vi "DFD Plot Phase Delay.vi"(4 "phase delay unit":u16(ring) items=["Samples", "Seconds"], 5 "output option":u16(ring) items=["Auto", "Floating-Point Only", "Fixed-Point Only"], 6 "fs [Hz]":dbl=-1.0 format="%.2f", 7 "# freq bins":i32=-1, 8 "error in (no error)":errorcluster, 11 "filter in":T1={"mSRate_Fs"=1.0, "mSRate_Version"="2.0", "mSRate_Comments"="", "mSRate_OrgCoef"={"type"=enum."Undefined", "gain"=1.0, "coef a (k)"=[], "coef b (v)"=[]}, "mSRate_CurCoef"={"type"=enum."Undefined", "gain"=1.0, "coef a (k)"=[], "coef b (v)"=[]}, "mSRate_Quantized?"=FALSE, "mSRate_QCoef"={"type"=enum."Undefined", "gain"=1.0, "coef a (k)"=[], "coef b (v)"=[]}, "mSRate_QSettings"=[], "mSRate_Order"=0, "mSRate_Scaling"={"mSRate_ScaleByPowerOf2?"=FALSE, "mSRate_ScaleType"=enum."No Norm"}} {"mSRate_QSettings"."source" items=["Coef a/k"=0, "Coef b/v"=7, "Input"=1, "Output"=2, "Multiplicand"=3, "Product"=4, "Sum"=5, "Delay"=6, "Gain"=8]}) -> (0 "error out":errorcluster, 2 "phase delay":cluster{"f0":dbl, "df":dbl, "values":dbl[]}[](graph), 3 "filter out":T1={"mSRate_Fs"=1.0, "mSRate_Version"="2.0", "mSRate_Comments"="", "mSRate_OrgCoef"={"type"=enum."Undefined", "gain"=1.0, "coef a (k)"=[], "coef b (v)"=[]}, "mSRate_CurCoef"={"type"=enum."Undefined", "gain"=1.0, "coef a (k)"=[], "coef b (v)"=[]}, "mSRate_Quantized?"=FALSE, "mSRate_QCoef"={"type"=enum."Undefined", "gain"=1.0, "coef a (k)"=[], "coef b (v)"=[]}, "mSRate_QSettings"=[], "mSRate_Order"=0, "mSRate_Scaling"={"mSRate_ScaleByPowerOf2?"=FALSE, "mSRate_ScaleType"=enum."No Norm"}} {"mSRate_QSettings"."source" items=["Coef a/k"=0, "Coef b/v"=7, "Input"=1, "Output"=2, "Multiplicand"=3, "Product"=4, "Sum"=5, "Delay"=6, "Gain"=8]})   [LabVIEW 2017, in "NI_DigFilterLicensed.lvlib"]
doc: "Plots the phase delay response of a filter."
uses:
  <vilib>/addons/Digital Filter Design/NI_DigFilterLicensed.lvlib
  <vilib>/addons/Digital Filter Design/_Objects.llb/DFD Filter Obj.ctl
  <vilib>/addons/Digital Filter Design/_Objects.llb/DFD Filter Coef.ctl
  <vilib>/addons/Digital Filter Design/_Objects.llb/DFD Filter Structure Type Selector.ctl
  <vilib>/addons/Digital Filter Design/_Objects.llb/dfd_Internal Quantization Settings.ctl
  <vilib>/addons/Digital Filter Design/_Objects.llb/dfd_Internal Quantization Srcs.ctl
  <vilib>/addons/Digital Filter Design/_Objects.llb/DFD Coef Norm Type.ctl
  <vilib>/addons/Digital Filter Design/_Objects.llb/DFD Phase Setting.ctl
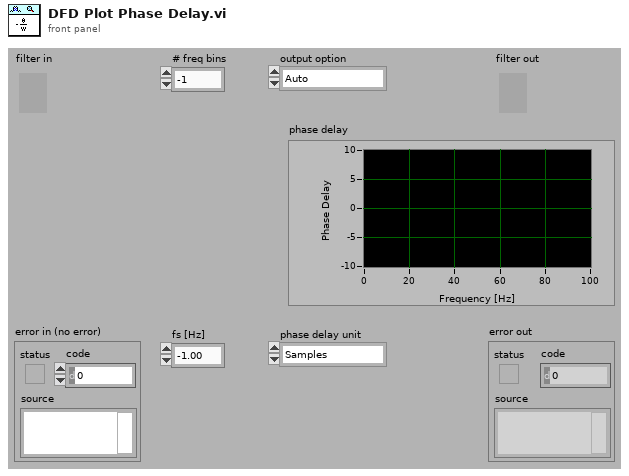
[diagram p1: front panel]
types:
  T1 = typedef "NI_DigFilterLicensed.lvlib/DFD Filter Obj.ctl" = cluster{"mSRate_Fs":dbl, "mSRate_Version":string, "mSRate_Comments":string, "mSRate_OrgCoef":T2, "mSRate_CurCoef":T2, "mSRate_Quantized?":bool, "mSRate_QCoef":T2, "mSRate_QSettings":T4[], "mSRate_Order":i32, "mSRate_Scaling":cluster{"mSRate_ScaleByPowerOf2?":bool, "mSRate_ScaleType":T6}}
  T2 = typedef "NI_DigFilterLicensed.lvlib/DFD Filter Coef.ctl" = cluster{"type":T3, "gain":dbl, "coef a (k)":dbl[], "coef b (v)":dbl[]}
  T3 = typedef "NI_DigFilterLicensed.lvlib/DFD Filter Structure Type Selector.ctl" = enum16{"Undefined", "FIR Direct Form", "FIR Direct Form Transposed", "FIR Symmetric", "FIR Antisymmetric", "IIR Direct Form I", "IIR Direct Form I Transposed", "IIR Direct Form II", "IIR Direct Form II Transposed", "IIR Cascaded Second Order Sections Form I", "IIR Cascaded Second Order Sections Form I Transposed", "IIR Cascaded Second Order Sections Form II", "IIR Cascaded Second Order Sections Form II Transposed", "Lattice Allpass (basic sections)", "Lattice Allpass (one multiplier sections)", "Lattice Allpass (normalized sections)", "Lattice AR (basic sections)", "Lattice AR (one multiplier sections)", "Lattice AR (normalized sections)", "Lattice MA (minimum phase)", "Lattice MA (maximum phase)", "Lattice ARMA (basic sections)", "Lattice ARMA (one multiplier sections)", "Lattice ARMA (normalized sections)"}
  T4 = typedef "NI_DigFilterLicensed.lvlib/dfd_Internal Quantization Settings.ctl" = cluster{"source":T5, "wl":i16, "iwl":i16, "overflow mode":enum16{"Saturation", "Wrap"}, "rounding mode":enum16{"Nearest", "Truncation"}, "signed?":bool}
  T5 = typedef "NI_DigFilterLicensed.lvlib/dfd_Internal Quantization Srcs.ctl" = u16
  T6 = typedef "NI_DigFilterLicensed.lvlib/DFD Coef Norm Type.ctl" = enum16{"No Norm", "Time Domain 1-Norm", "Time Domain 2-Norm", "Time Domain Inf-Norm"}
  T7 = typedef "NI_DigFilterLicensed.lvlib/DFD Phase Setting.ctl" = cluster{"unwrap? (F)":bool, "degree? (F)":bool}
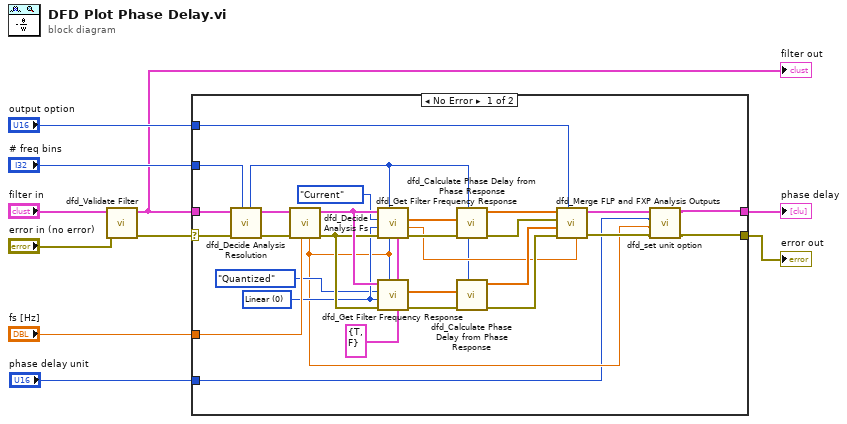
[diagram p0: block diagram]
diagram:
  n1 = call <vilib>:"dfd_Validate Filter.vi"("error in (no error)"="error in (no error)", "filter in"="filter in") -> ("error out"=w3:errorcluster, "filter out"=w4:T1)  [unwired: 1 in, 7 out]
  "filter out" <- w4
  n2 = case shown="No Error" w3 {
    selector: w3 -> [w36 w40]
    tunnel: "# freq bins" -> [w38 _]
    tunnel: w4 -> [w37 _]
    tunnel: "fs [Hz]" -> [w39 _]
    tunnel: [w14 w40] -> w6
    tunnel: "output option" -> [w33 _]
    tunnel: [w15 _] -> w7
    tunnel: "phase delay unit" -> [w11 _]
    frame No Error {
      w19 = u16 0 items=["Linear", "dB", "Zero phase"] ("magnitude")
      w20 = T7 {"unwrap? (F)"=TRUE, "degree? (F)"=FALSE} ("phase view")
      n3 = call <vilib>:"dfd_Decide Analysis Resolution.vi"("# freq bins in"=w38, "error in (no error)"=w36, "filter in"=w37) -> ("error out"=w35:errorcluster, "filter out"=w34:T1, "# freq bins out"=w21:i32)  [unwired: 3 in, 3 out]
      n4 = call <vilib>:"dfd_Decide Analysis Fs.vi"("fs in [Hz]"=w39, "error in (no error)"=w35, "filter in"=w34) -> ("error out"=w24:errorcluster, "filter out"=w26:T1, "fs out [Hz]"=w12:dbl)  [unwired: 1 in, 5 out]
      n5 = call <vilib>:"dfd_Get Filter Frequency Response.vi"("phase view"=w20, "fs [Hz]"=w12, "# freq bins"=w21, "error in (no error)"=w24, "magnitude"=w19, "coef source"=enum16{"Original", "Current", "Quantized"}."Current", "filter in"=w26) -> ("error out"=w27:errorcluster, "df"=w22:dbl, "phase"=w28:dbl[])  [unwired: 2 out]
      n6 = call <vilib>:"dfd_Get Filter Frequency Response.vi"("phase view"=w20, "fs [Hz]"=w12, "# freq bins"=w21, "error in (no error)"=w24, "magnitude"=w19, "coef source"=enum16{"Original", "Current", "Quantized"}."Quantized", "filter in"=w26) -> ("error out"=w23:errorcluster, "phase"=w25:dbl[])  [unwired: 3 out]
      n7 = call <vilib>:"dfd_Calculate Phase Delay from Phase Response.vi"("#freq bins"=w21, "error in (no error)"=w27, "phase"=w28) -> ("error out"=w30:errorcluster, "phase delay"=w32:dbl[])  [unwired: 1 in, 6 out]
      n8 = call <vilib>:"dfd_Calculate Phase Delay from Phase Response.vi"("#freq bins"=w21, "error in (no error)"=w23, "phase"=w25) -> ("error out"=w29:errorcluster, "phase delay"=w31:dbl[])  [unwired: 2 in, 5 out]
      n9 = call <vilib>:"dfd_Merge FLP and FXP Analysis Outputs.vi"("delta"=w22, "output option"=w33, "error in FXP"=w29, "response FXP"=w31, "error in FLP"=w30, "response FLP"=w32) -> ("error out"=w13:errorcluster, "freq responses"=w16:cluster{"f0":dbl, "df":dbl, "values":dbl[]}[])  [unwired: 4 out]
      n10 = call <vilib>:"dfd_set unit option.vi"("error in (no error)"=w13, "fs [Hz]"=w12, "unit option"=w11, "freq responses"=w16) -> ("error out"=w14:errorcluster, "freq responses out"=w15:cluster{"f0":dbl, "df":dbl, "values":dbl[]}[])  [unwired: 6 out]
    }
    frame Error {
    }
  }
  "error out" <- w6
  "phase delay" <- w7
